vi "Pop.vi"(3 "Error In":errorcluster, 4 "Delete?":bool, 5 "object in":refnum<class "Stack.lvclass">) -> (0 "Error Out":errorcluster, 1 "Data":variant, 2 "object out":refnum<class "Stack.lvclass">)   [LabVIEW 2024, in "Stack.lvclass"]
uses:
  Stack.lvclass
  Stack.lvclass/Stack.ctl
panel:
  # "Connector Pane"
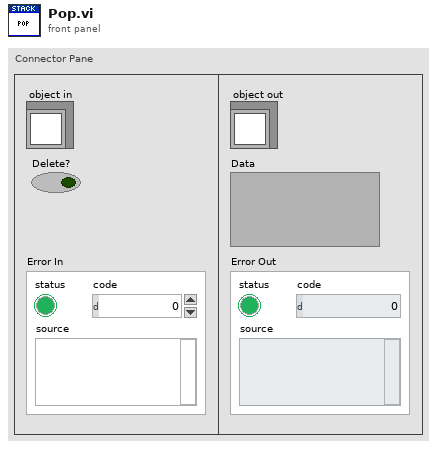
[diagram p1: front panel]
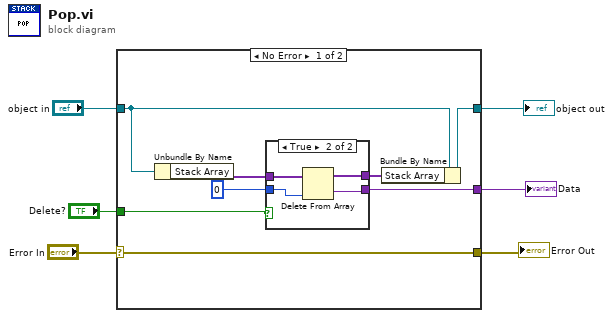
[diagram p0: block diagram]
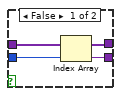
[diagram p2: hidden frame]
diagram:
  n1 = case shown="No Error" "Error In" {
    selector: "Error In" -> [w14 w23]
    tunnel: [w14 w23] -> w5
    tunnel: [w9 w22] -> w3
    tunnel: "object in" -> [w13 w22]
    tunnel: [w10 _] -> w2
    tunnel: "Delete?" -> [w7 _]
    frame No Error {
      n2 = Unbundle By Name(w13) -> ("Stack Array"=w12:variant[])
      n3 = case shown="True" w7 {
        tunnel: w12 -> [w15 w21]
        tunnel: 0 ("index") -> [w17 w20]
        tunnel: [w16 w19] -> w10
        tunnel: [w15 w18] -> w8
        frame False {
          n4 = Index Array(array=w15, index=w17) -> (element=w16:variant)
        }
        frame True {
          n5 = Delete From Array(array=w21, index=w20) -> (deleted portion=w19:variant, array with subset deleted=w18:variant[])  [unwired: 1 in]
        }
      }
      n6 = Bundle By Name(cluster=w13, "Stack Array"=w8) -> (w9:refnum<class "Stack.lvclass">)
    }
    frame Error {
    }
  }
  "Error Out" <- w5
  "object out" <- w3
  "Data" <- w2
